vi "Self Test.vi"(8 "error in":errorcluster, 11 "69X_79X in":refnum<class "7976A.lvclass">) -> (0 "error out":errorcluster, 3 "69X_79X out":refnum<class "7976A.lvclass">)   [LabVIEW 2019, in "7976A.lvlib" / "7976A.lvclass"]
uses:
  Library/7976A.lvclass
  Library/7976A.lvclass/7976A.ctl
  builds/Instruments/PowerSupply.lvlibp/Library/PowerSupply.lvclass
  <instrlib>/Agilent N7976A/Agilent N7976A.lvlib
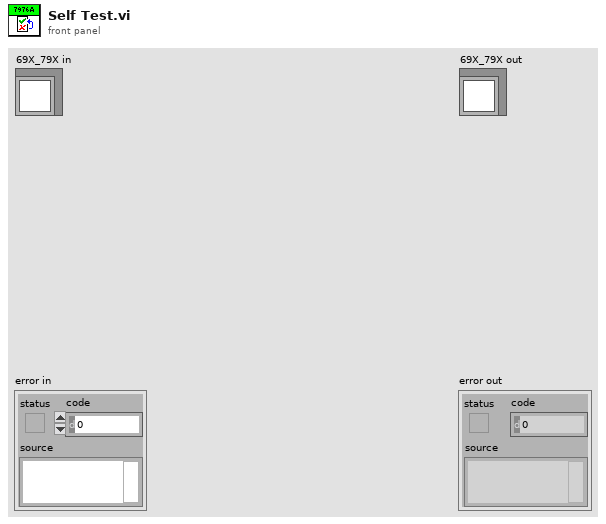
[diagram p1: front panel]
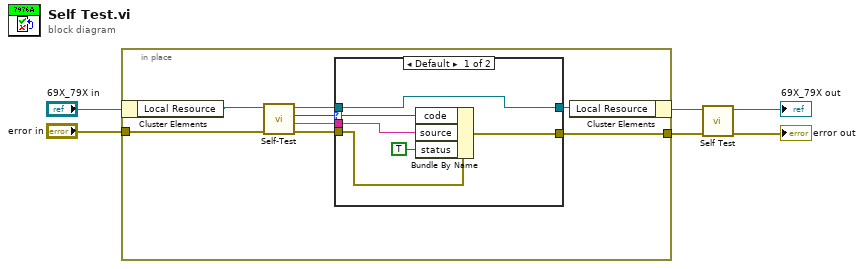
[diagram p0: block diagram]
diagram:
  n1 = in-place {
    in-place-border: "error in" -> [w10]
    in-place-border: [w13] -> w2
    n2 = in-place-cluster #1("69X_79X in") -> ("Local Resource"=w12:refnum<visa-resource-name>)
    n3 = call <instrlib>:"Self-Test.vi"("error in (no error)"=w10, "VISA resource name"=w12) -> ("error out"=w9:errorcluster, "Self-Test Result Message"=w8:string, "Self-Test Result Code"=w7:i32, "VISA resource name out"=w11:refnum<visa-resource-name>)  [unwired: 6 in]
    n4 = case shown="Default" w7 {
      selector: w7 -> [w19 _]
      tunnel: w11 -> [w15 w21]
      tunnel: w9 -> [w20 w22]
      tunnel: w8 -> [w18 _]
      tunnel: [w16 w22] -> w13
      tunnel: [w15 w21] -> w14
      frame Default {
        n5 = Bundle By Name(cluster=w20, "code"=w19, "source"=w18, "status"=TRUE) -> (w16:errorcluster)
      }
      frame 0 {
      }
    }
    n6 = in-place-cluster #1("Local Resource"=w14) -> (w4:refnum<class "7976A.lvclass">)
  }
  n7 = call-parent "Self Test.vi"("error in"=w2, "Instruments in"=w4) -> ("error out"=→"error out":errorcluster, "Instruments out"=→"69X_79X out":refnum<class "7976A.lvclass">)  [unwired: 8 in]
